vi "Close.vi"(8 "error in":errorcluster, 11 "Cell Context in":refnum<class "Cell Context.lvclass">) -> (0 "error out":errorcluster, 3 "Cell Context out":refnum<class "Cell Context.lvclass">)   [LabVIEW 2023, in "SourceGrid.lvlib" / "Cell Context.lvclass"]
uses:
  Cell Context.lvclass
  Cell Context.lvclass/Cell Context.ctl
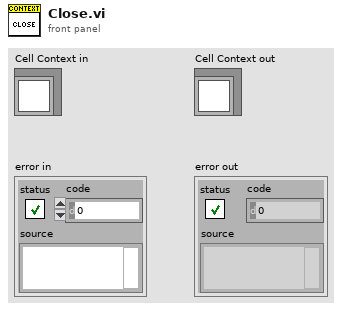
[diagram p1: front panel]
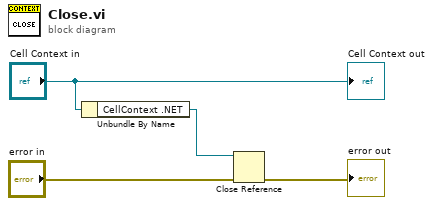
[diagram p0: block diagram]
diagram:
  n1 = Unbundle By Name("Cell Context in") -> ("CellContext .NET"=w1:refnum<k24>)
  n2 = Close Reference(reference=w1, error in (no error)="error in") -> (error out=→"error out":errorcluster)
  "Cell Context out" <- "Cell Context in"
